vi "Generador_DAQ_Continuas.vi"() -> ()   [LabVIEW 2015]
uses:
  <vilib>/DAQmx/write.llb/DAQmx Write (Analog 1D DBL 1Chan NSamp).vi
  <vilib>/DAQmx/create/channels.llb/DAQmx Create Channel (AO-Voltage-Basic).vi
  <vilib>/DAQmx/configure/timing.llb/DAQmx Timing (Sample Clock).vi
  <vilib>/DAQmx/miscellaneous.llb/DAQmx Fill In Error Info.vi
panel:
  in  "stop":bool
  out "Waveform Graph":dbl[](graph)
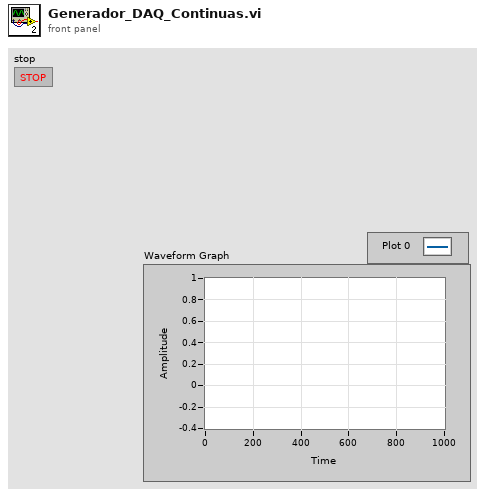
[diagram p1: front panel]
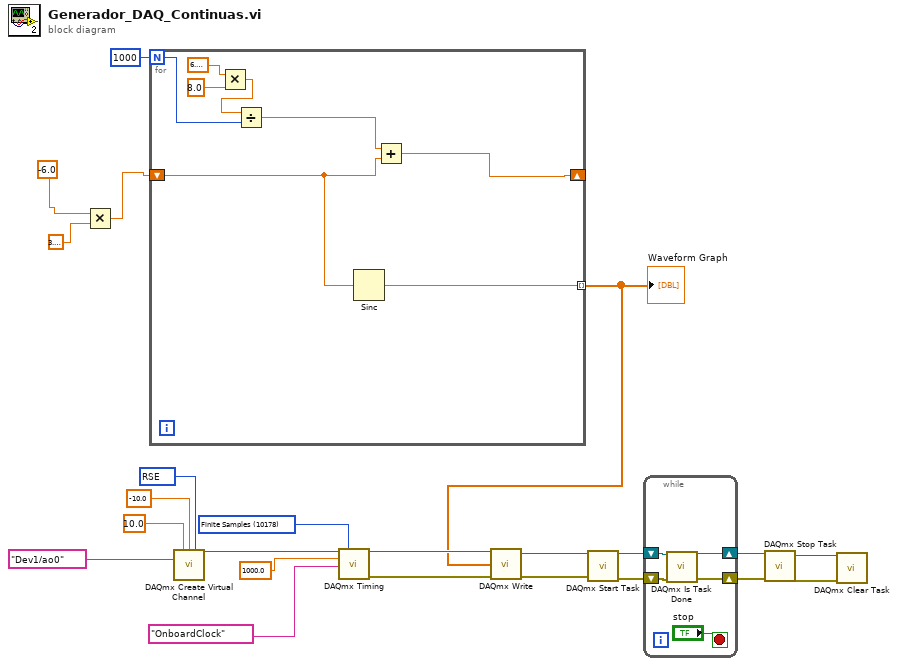
[diagram p0: block diagram]
diagram:
  w17 = 10178 items=["Finite Samples"=10178, "Continuous Samples"=10123, "Hardware Timed Single Point"=12522] ("sample mode")
  w22 = 10083 items=["Default"=-1, "RSE"=10083, "Differential"=10106, "Pseudodifferential"=12529] ("output terminal configuration")
  n1 = Multiply(x=-6.0, y=3.141592653589793) -> (x*y=w11:dbl)
  n2 = for {
    N: 1000 -> [w31]
    shift-right: [w29] -> _
    shift-left: w11 -> [w28]
    tunnel: [w27] -> w12 mode=indexing
    n3 = Multiply(x=6.283185307179586, y=8.0) -> (x*y=w24:dbl)
    n4 = Divide(x=w24, y=w31) -> (x/y=w30:dbl)
    n5 = Sinc(1:w28) -> (0:w27:dbl)
    n6 = Add(x=w30, y=w28) -> (x+y=w29:dbl)
  }
  "Waveform Graph" <- w12
  n7 = call-poly <vilib>:"DAQmx Create Virtual Channel.vi"("maximum value"=10.0, "minimum value"=-10.0, "output terminal configuration"=w22, "physical channels"=tag "Dev1/ao0") -> ("task out"=w19:refnum<k21>)  [unwired: 10 in, 1 out]
  n8 = call-poly <vilib>:"DAQmx Timing.vi"("task/channels in"=w19, "sample mode"=w17, "rate"=1000.0, "source"=tag "OnboardClock") -> ("task out"=w14:refnum<k21>, "error out"=w13:errorcluster)  [unwired: 10 in]
  n9 = call-poly <vilib>:"DAQmx Write.vi"("task/channels in"=w14, "data"=w12, "error in"=w13) -> ("task out"=w6:refnum<k21>, "error out"=w5:errorcluster)  [unwired: 10 in, 1 out]
  n10 = call <vilib>:"DAQmx Start Task.vi"("task/channels in"=w6, "error in"=w5) -> ("task out"=w4:refnum<k21>, "error out"=w3:errorcluster)  [unwired: 12 in]
  n11 = while {
    shift-right: [w33] -> w1
    shift-left: w4 -> [w36]
    shift-right: [w34] -> w2
    shift-left: w3 -> [w35]
    stop <- "stop" stop-if-true
    n12 = call <vilib>:"DAQmx Is Task Done.vi"("task/channels in"=w36, "error in"=w35) -> ("task out"=w33:refnum<k21>, "error out"=w34:errorcluster)  [unwired: 11 in, 1 out]
  }
  n13 = call <vilib>:"DAQmx Stop Task.vi"("task/channels in"=w1, "error in"=w2) -> ("task out"=w8:refnum<k21>, "error out"=w7:errorcluster)  [unwired: 12 in]
  n14 = call <vilib>:"DAQmx Clear Task.vi"("task in"=w8, "error in"=w7) -> ()  [unwired: 13 in, 1 out]
